vi "Enable_Disable Batch.vi"(8 "error in (no error)":errorcluster, 9 "Enable (T)":bool, 10 "Control Names":string[](array[string]), 11 "Controls_Mgr in":refnum<class "Controls_Mgr.lvclass">) -> (0 "error out":errorcluster, 3 "Controls_Mgr out":refnum<class "Controls_Mgr.lvclass">)   [LabVIEW 2015, in "Generic Module Library.lvlib" / "Template G_Module.lvlib" / "Controls_Mgr.lvclass"]
uses:
  Controls_Mgr.lvclass
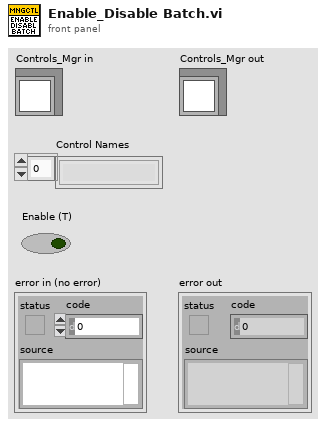
[diagram p1: front panel]
types:
  T1 = enum8{"Enabled", "Disabled", "Disabled and Grayed Out"}
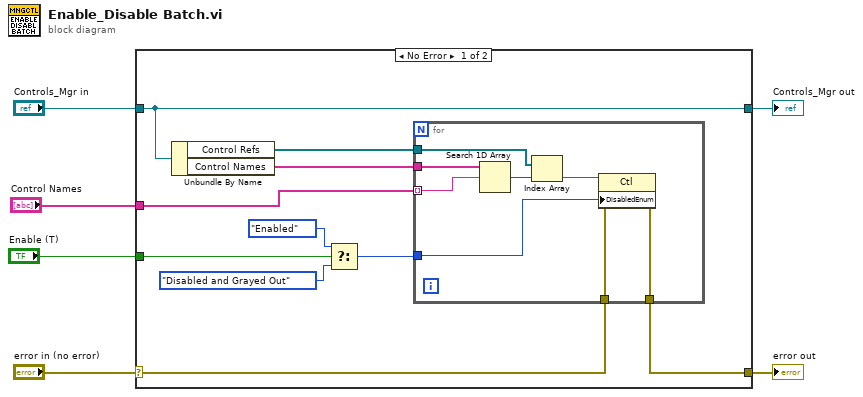
[diagram p0: block diagram]
diagram:
  n1 = case shown="No Error" "error in (no error)" {
    selector: "error in (no error)" -> [w11 w26]
    tunnel: [w10 w26] -> w5
    tunnel: [w13 w25] -> w3
    tunnel: "Controls_Mgr in" -> [w13 w25]
    tunnel: "Control Names" -> [w14 _]
    tunnel: "Enable (T)" -> [w8 _]
    frame No Error {
      n2 = Unbundle By Name(w13) -> ("Control Refs"=w16:refnum<vi>[], "Control Names"=w15:string[])
      n3 = Select(t=T1."Enabled" ("Disabled"), s=w8, f=T1."Disabled and Grayed Out" ("Disabled")) -> (s? t:f=w7:T1)
      n4 = for {
        tunnel: w16 -> [w23]
        tunnel: w15 -> [w22]
        tunnel: w14 -> [w21] mode=indexing
        tunnel: w11 -> [w19]
        tunnel: [w18] -> w10
        tunnel: w7 -> [w17]
        n5 = Search 1D Array(1D array=w22, element=w21) -> (index of element=w24:i32)  [unwired: 1 in]
        n6 = Index Array(array=w23, index=w24) -> (element=w20:refnum<vi>)
        n7 = property class="Ctl"(reference=w20, error in=w19, "DisabledEnum"=w17) -> (error out=w18:errorcluster)  [unwired: 1 out]
      }
    }
    frame Error {
    }
  }
  "error out" <- w5
  "Controls_Mgr out" <- w3
